vi "Actividad 2-Calculadora.vi"() -> ()   [LabVIEW 2018]
panel:
  in  "stop":bool
  out "String":string
  in  "borrar":bool
  in  "division":bool
  in  "igual":bool
  in  "punto":bool
  in  "0":bool
  in  "multiplicacion":bool
  in  "tres":bool
  in  "dos":bool
  in  "uno":bool
  in  "resta":bool
  in  "seis":bool
  in  "cinco":bool
  in  "cuatro":bool
  in  "suma":bool
  in  "nueve":bool
  in  "ocho":bool
  in  "siete":bool
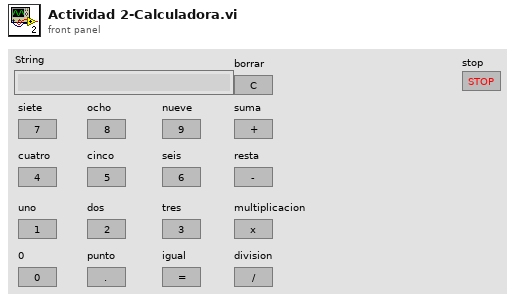
[diagram p1: front panel]
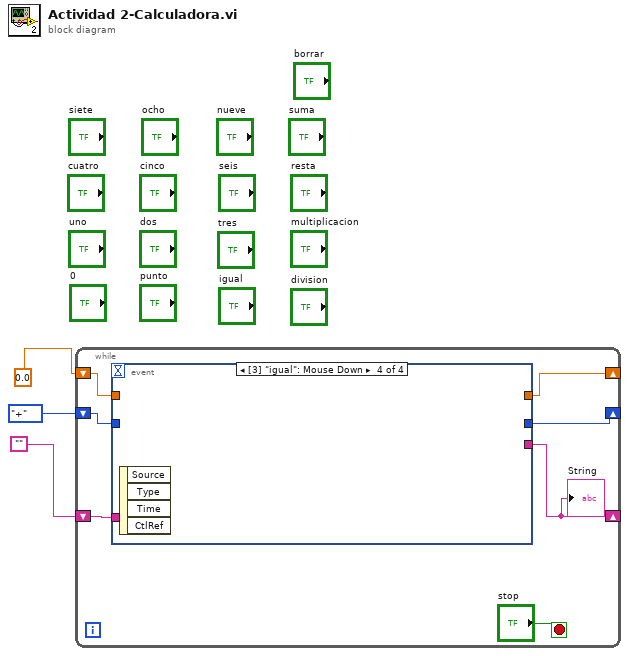
[diagram p0: block diagram]
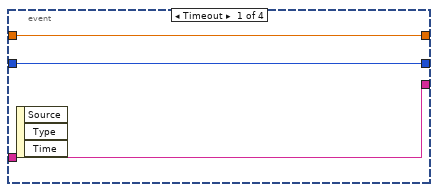
[diagram p2: hidden frame]
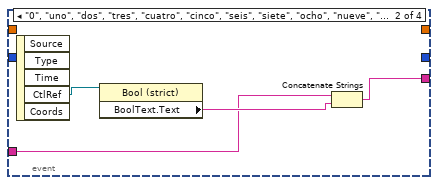
[diagram p3: hidden frame]
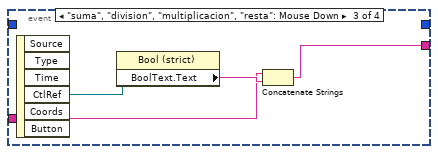
[diagram p4: hidden frame]
diagram:
  n1 = while {
    shift-right: [w8] -> _
    shift-left: 0.0 -> [w9]
    shift-right: [w6] -> _
    shift-left: enum16{"+", "-", "x", "/"}."+" -> [w7]
    shift-right: [w4] -> _
    shift-left: "" -> [w5]
    stop <- "stop" stop-if-true
    n2 = event shown="[3] \"igual\": Mouse Down" {
      selector: _ -> [_ _ _ _]
      dyn-events: _ -> [_ _ _ _]
      timeout: _ -> [_ _ _ _]
      tunnel: w9 -> [w13 _ _ _]
      tunnel: [w13 _ _ _] -> w8
      tunnel: w7 -> [w12 _ _ _]
      tunnel: [w12 _ _ _] -> w6
      tunnel: w5 -> [w11 w16 w19 _]
      tunnel: [w11 w15 w18 _] -> w4
      event Timeout {
        n3 = event-data() -> ()  [unwired: 1 in, 3 out]
      }
      event "0", "uno", "dos", "tres", "cuatro", "cinco", "seis", "siete", "ocho", "nueve", "punto": Mouse Down {
        n4 = event-data() -> ("CtlRef"=w14:refnum<vi>)  [unwired: 1 in, 4 out]
        n5 = property class="Bool (strict)"(reference=w14) -> ("BoolText.Text"=w17:string)  [unwired: 1 in, 2 out]
        n6 = Concatenate Strings(w16, w17) -> (w15:string)
      }
      event "suma", "division", "multiplicacion", "resta": Mouse Down {
        n7 = event-data() -> ("CtlRef"=w21:refnum<vi>)  [unwired: 1 in, 5 out]
        n8 = property class="Bool (strict)"(reference=w21) -> ("BoolText.Text"=w20:string)  [unwired: 1 in, 2 out]
        n9 = Concatenate Strings(w19, w20) -> (w18:string)
      }
      event "igual": Mouse Down {
        n10 = event-data() -> ()  [unwired: 1 in, 4 out]
      }
    }
    "String" <- w4
  }
